vi "destroy.vi"(8 "error in (no error)":errorcluster, 11 "ExampleTask_StopNotifier in":refnum<class "Task_BoolStopNotifier.lvclass">) -> (0 "error out":errorcluster, 3 "loopCounter":i32)   [LabVIEW 2023, in "Task_BoolStopNotifier.lvclass"]
doc: "Destructor.\nIt also returns the value of loopCounter."
uses:
  Task_BoolStopNotifier.lvclass
  Task_BoolStopNotifier.lvclass/Task_BoolStopNotifier.ctl
  Read loopCounter.vi
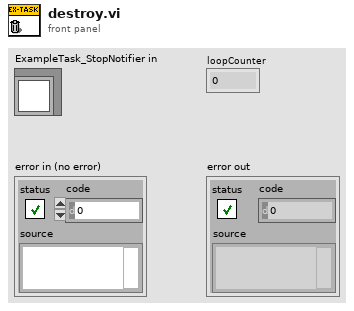
[diagram p1: front panel]
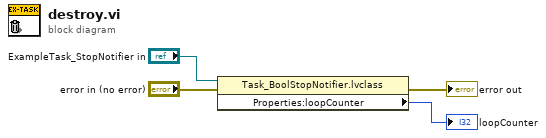
[diagram p0: block diagram]
diagram:
  n1 = property class="Task_BoolStopNotifier.lvclass"(reference="ExampleTask_StopNotifier in", error in="error in (no error)") -> (error out=→"error out":errorcluster, "Properties:loopCounter"=→"loopCounter":i32)  [unwired: 1 out]
